vi "get_price.vi"(8 "error in (no error)":errorcluster, 11 "Table in":refnum<class "Table.lvclass">) -> (0 "error out":errorcluster, 2 "price":dbl, 3 "Table out":refnum<class "Table.lvclass">)   [LabVIEW 2021, in "Table.lvclass"]
uses:
  Table.lvclass
  Table.lvclass/Table.ctl
  1a15e72c-6628-3fec-b06d-93136bedeb3f.vi
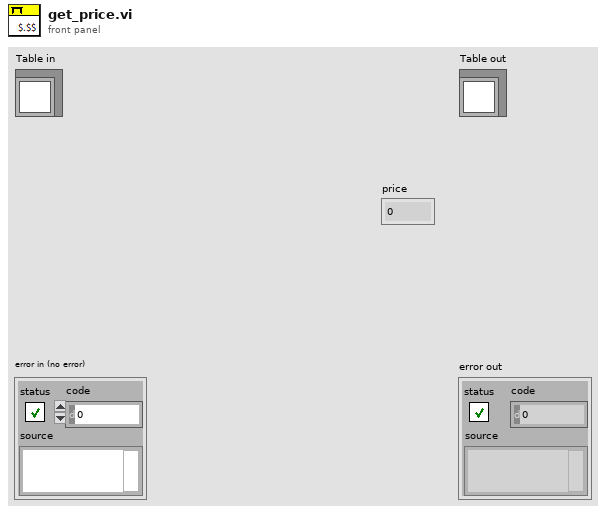
[diagram p1: front panel]
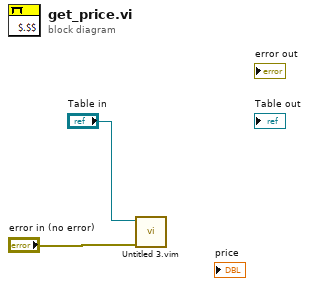
[diagram p0: block diagram]
diagram:
  n1 = call "Untitled 3.vim"("Table in"="Table in", "error in (no error)"="error in (no error)") -> ()  [unwired: 6 in, 3 out]
